vi "Resolve Path.vi"(1 "Starting Path":path, 2 "Path":path) -> (0 "Resolved Path":path)   [LabVIEW 2020, in "Volatus.lvlib"]
uses:
  Volatus Core/Volatus Core.lvclass/Volatus Core.ctl
  Volatus.lvlib
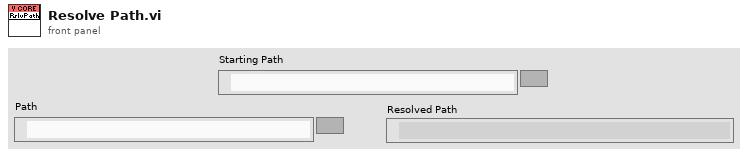
[diagram p1: front panel]
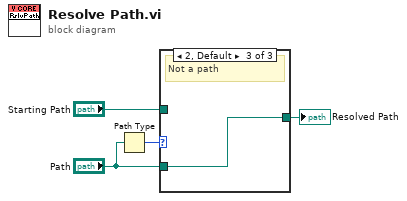
[diagram p0: block diagram]
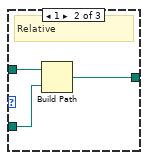
[diagram p3: hidden frame]
diagram:
  n1 = Path Type(1:"Path") -> (0:w4:i16)
  n2 = case shown="2, Default" w4 {
    tunnel: "Starting Path" -> [_ w8 _]
    tunnel: "Path" -> [w5 w7 w9]
    tunnel: [w5 w6 w9] -> w1
    frame 0 {
      # "Absolute"
    }
    frame 1 {
      # "Relative"
      n3 = Build Path(base path=w8, name or relative path=w7) -> (appended path=w6:path)
    }
    frame 2, Default {
      # "Not a path"
    }
  }
  "Resolved Path" <- w1
